vi "Teleop.vi"(10 "Match Info":T1={"Autonomous Elapsed Seconds"=0.0, "TeleOp Elapsed Seconds"=0.0, "Disabled Elapsed Seconds"=0.0, "Visited Autonomous"=FALSE, "Visited TeleOp"=FALSE, "Visited Disabled"=FALSE, "Autonomous Settings"={"Autonomous Style"=enum."Independent", "VI Refnum"=refnum}}, 11 "Call Context":T2) -> ()   [LabVIEW 2016]
doc: "This VI is called for each TeleOp packet received from the DS where the robot is not disabled. It is often used to read from the joysticks and update I/O or to update setpoints for timed control loops. It should complete and return within 20 milliseconds or it may miss DS packets."
uses:
  <vilib>/Rock Robotics/WPI/DriverStation/WPI_DriverStationDerivedRobotMode.ctl
  <vilib>/Rock Robotics/WPI/DriverStation/WPI_DriverStationMatch Info.ctl
  <vilib>/Rock Robotics/WPI/Solenoid/WPI_SolenoidValue.ctl
  <vilib>/Rock Robotics/WPI/ThirdParty/CanMotor/CTRLib-LV-TalonSRX/CTRE_CANTalonSRX_ControlMode.ctl
  <vilib>/Rock Robotics/WPI/Utilities/WPI_GetSetVariantRefNum.vi
  <vilib>/Rock Robotics/Network Tables/NT Write Boolean Array.vi
  <vilib>/Rock Robotics/Network Tables/NT Write Numeric Array.vi
  <vilib>/Rock Robotics/Network Tables/NT Read Boolean.vi
  <vilib>/Rock Robotics/Network Tables/NT Read Number.vi
  <vilib>/Rock Robotics/WPI/Solenoid/WPI_SolenoidSetEnum.vi
panel:
  out "Sample Slider 0":dbl(slide) scale=0.0..5.0
  out "Sample Boolean 1":bool
  out "Sample Boolean 0":bool
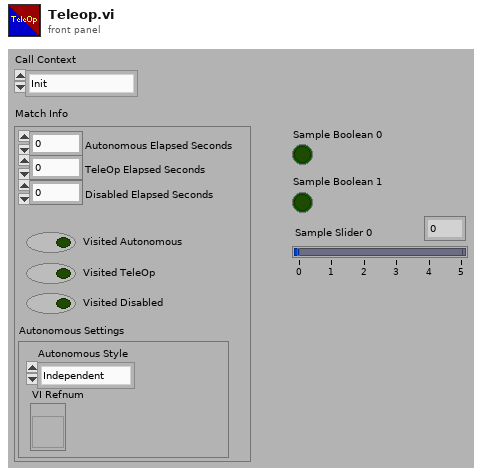
[diagram p1: front panel]
types:
  T1 = typedef "WPI_DriverStationMatch Info.ctl" = cluster{"Autonomous Elapsed Seconds":dbl, "TeleOp Elapsed Seconds":dbl, "Disabled Elapsed Seconds":dbl, "Visited Autonomous":bool, "Visited TeleOp":bool, "Visited Disabled":bool, "Autonomous Settings":cluster{"Autonomous Style":enum16{"Iterative", "Independent"}, "VI Refnum":refnum<vi>}}
  T2 = typedef "WPI_DriverStationDerivedRobotMode.ctl" = enum16{"Init", "Execute", "Stop"}
  T3 = typedef "CTRE_CANTalonSRX_ControlMode.ctl" = enum16{"Throttle (Duty-Cycle)", "Position Closed-Loop", "Velocity Closed-Loop", "Current Closed-Loop", "Voltage Compensation", "Slave Follower", "Motion Profile", "Motion Magic"}
  T4 = typedef "WPI_MotorControlDeviceRef.ctl" = cluster{"DeviceStatus":errorcluster, "Type":T5, "PWM":cluster{"PWM Channel":T6, "DeadBand":T7}, "CAN":cluster{"Device Number":u8, "SetOutput VI Ref":variant, "GetOutput VI Ref":variant, "Enable VI Ref":variant, "Disable VI Ref":variant, "Data":variant}, "Invert":bool}
  T5 = typedef "WPI_MotorControlType.ctl" = enum16{"PWM", "CAN"}
  T6 = typedef "FPGA_DIOPWMChannel.ctl" = enum8{"PWM 0", "PWM 1", "PWM 2", "PWM 3", "PWM 4", "PWM 5", "PWM 6", "PWM 7", "PWM 8", "PWM 9", "PWM MXP 0", "PWM MXP 1", "PWM MXP 2", "PWM MXP 3", "PWM MXP 4", "PWM MXP 5", "PWM MXP 6", "PWM MXP 7", "PWM MXP 8", "PWM MXP 9", "Invalid"}
  T7 = typedef "WPI_PWMDeadband.ctl" = cluster{"Name":string, "maxPositivePwm":i32, "minPositivePwm":i32, "centerPwm":i32, "maxNegativePwm":i32, "minNegativePwm":i32, "angularRange":u16}
  T8 = typedef "WPI_JoystickDevRef.ctl" = cluster{"Device":T9}
  T9 = typedef "WPI_JoystickDeviceEnum.ctl" = enum16{"USB 0", "USB 1", "USB 2", "USB 3", "USB 4", "USB 5"}
  T10 = cluster{"Axes[0]":dbl, "Axes[1]":dbl, "Axes[2]":dbl, "Axes[3]":dbl, "Axes[4]":dbl, "Axes[5]":dbl, "Axes[6]":dbl, "Axes[7]":dbl, "Axes[8]":dbl}
  T11 = cluster{"Buttons[0]":bool, "Buttons[1]":bool, "Buttons[2]":bool, "Buttons[3]":bool, "Buttons[4]":bool, "Buttons[5]":bool, "Buttons[6]":bool, "Buttons[7]":bool, "Buttons[8]":bool}
  T12 = cluster{"POVs[0]":i16, "POVs[1]":i16, "POVs[2]":i16, "POVs[3]":i16, "POVs[4]":i16, "POVs[5]":i16, "POVs[6]":i16, "POVs[7]":i16, "POVs[8]":i16}
  T13 = typedef "WPI_SolenoidDevRef.ctl" = cluster{"DevStatus":errorcluster, "Pneumatics Control Module":u8, "Forward Solenoid Channel":T14, "Reverse Solenoid Channel":T14}
  T14 = typedef "WPI_SolenoidChannel.ctl" = enum8{"Solenoid 0", "Solenoid 1", "Solenoid 2", "Solenoid 3", "Solenoid 4", "Solenoid 5", "Solenoid 6", "Solenoid 7", "Invalid"}
  T15 = typedef "WPI_SolenoidValue.ctl" = enum16{"Off", "On", "Forward", "Reverse"}
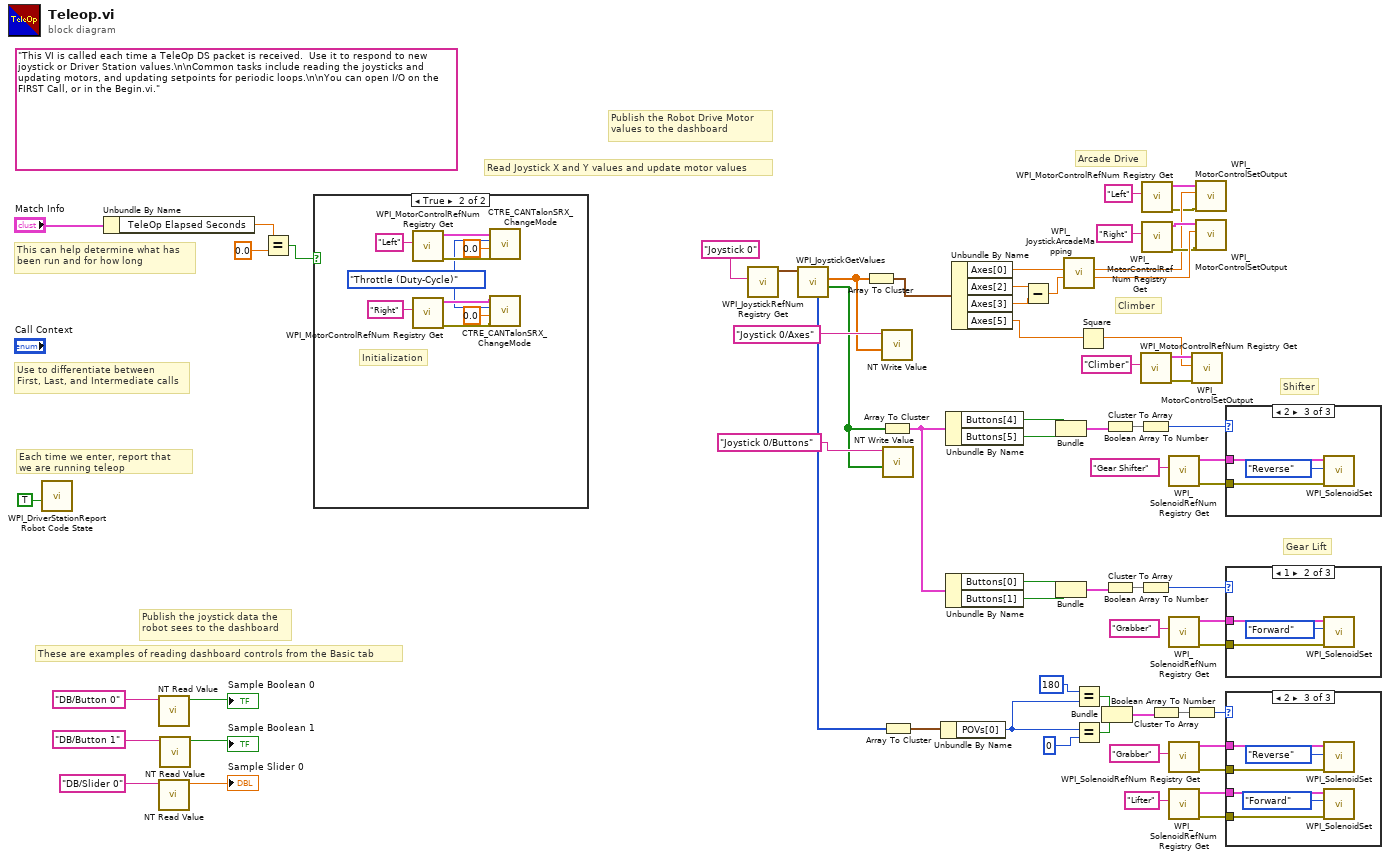
[diagram p0: block diagram]
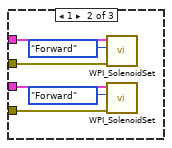
[diagram p3: hidden frame]
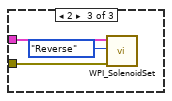
[diagram p5: hidden frame]
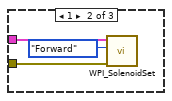
[diagram p7: hidden frame]
diagram:
  (unwired) "This VI is called each time a TeleOp DS packet is received.  Use it to respond to new joystick or Driver Station values.\n\nCommon tasks include reading the joysticks and updating motors, and updating setpoints for periodic loops.\n\nYou can open I/O on the FIRST Call, or in the Begin.vi."
  # "Gear Lift"
  # "Shifter"
  # "Climber"
  # "Arcade Drive"
  # "These are examples of reading dashboard controls from the Basic tab"
  # "Publish the Robot Drive Motor\nvalues to the dashboard"
  # "Publish the joystick data the\nrobot sees to the dashboard"
  # "Each time we enter, report that\nwe are running teleop"
  # "Use to differentiate between\nFirst, Last, and Intermediate calls"
  # "This can help determine what has\nbeen run and for how long"
  # "Read Joystick X and Y values and update motor values"
  n1 = call <vilib>:"WPI_DriverStationReport Robot Code State.vi"("TeleOp"=TRUE ("Autonomous")) -> ()  [unwired: 10 in, 1 out]
  n2 = Unbundle By Name("Match Info") -> ("TeleOp Elapsed Seconds"=w39:dbl)
  n3 = call-poly <vilib>:"NT Read Value.vi"("Name"="DB/Button 0" ("refnum name")) -> ("Boolean"=→"Sample Boolean 0":bool)  [unwired: 9 in, 1 out]
  n4 = call-poly <vilib>:"NT Read Value.vi"("Name"="DB/Slider 0" ("refnum name")) -> ("Numeric"=→"Sample Slider 0":dbl)  [unwired: 9 in, 1 out]
  n5 = call-poly <vilib>:"NT Read Value.vi"("Name"="DB/Button 1" ("refnum name")) -> ("Boolean"=→"Sample Boolean 1":bool)  [unwired: 9 in, 1 out]
  n6 = Equal?(x=w39, y=0.0) -> (x = y?=w38:bool)
  n7 = case shown="True" w38 {
    frame False {
    }
    frame True {
      w71 = CTRE_CANTalonSRX_ControlMode."Throttle (Duty-Cycle)" ("Talon SRX Control Mode")
      # "Initialization"
      n8 = call <vilib>:"WPI_MotorControlRefNum Registry Get.vi"("refnum name"="Left") -> ("error out"=w73:errorcluster, "MotorControlDevRef"=w74:T4)  [unwired: 9 in]
      n9 = call <vilib>:"WPI_MotorControlRefNum Registry Get.vi"("refnum name"="Right") -> ("error out"=w72:errorcluster, "MotorControlDevRef"=w75:T4)  [unwired: 9 in]
      n10 = call <vilib>:"CTRE_CANTalonSRX_ChangeMode.vi"("error in (no error)"=w73, "Output"=0.0, "Talon SRX Control Mode"=w71, "CAN Talon SRX Ref"=w74) -> ()  [unwired: 6 in, 2 out]
      n11 = call <vilib>:"CTRE_CANTalonSRX_ChangeMode.vi"("error in (no error)"=w72, "Output"=0.0, "Talon SRX Control Mode"=w71, "CAN Talon SRX Ref"=w75) -> ()  [unwired: 6 in, 2 out]
    }
  }
  n12 = call <vilib>:"WPI_JoystickRefNum Registry Get.vi"("refnum name"="Joystick 0") -> ("JoystickDevRef"=w66:T8)  [unwired: 1 in, 9 out]
  n13 = call <vilib>:"WPI_JoystickGetValues.vi"("JoystickDevRef"=w66) -> ("Buttons"=w56:bool[], "Axes"=w54:dbl[], "POVs"=w55:i16[])  [unwired: 6 in, 2 out]
  n14 = Array To Cluster(array=w54) -> (cluster=w53:T10)
  n15 = call-poly <vilib>:"NT Write Value.vi"("Numeric Array"=w54, "Name"="Joystick 0/Axes") -> ()  [unwired: 9 in, 1 out]
  n16 = Array To Cluster(array=w56) -> (cluster=w20:T11)
  n17 = call-poly <vilib>:"NT Write Value.vi"("Boolean Array"=w56, "Name"="Joystick 0/Buttons") -> ()  [unwired: 9 in, 1 out]
  n18 = Array To Cluster(array=w55) -> (cluster=w52:T12)
  n19 = Unbundle By Name(w52) -> ("POVs[0]"=w23:i16)
  n20 = Unbundle By Name(w20) -> ("Buttons[4]"=w31:bool, "Buttons[5]"=w30:bool)
  n21 = Unbundle By Name(w20) -> ("Buttons[0]"=w13:bool, "Buttons[1]"=w12:bool)
  n22 = Unbundle By Name(w53) -> ("Axes[0]"=w37:dbl, "Axes[2]"=w49:dbl, "Axes[3]"=w48:dbl, "Axes[5]"=w33:dbl)
  n23 = Subtract(x=w49, y=w48) -> (x-y=w47:dbl)
  n24 = Bundle("Buttons[4]"=w31, "Buttons[5]"=w30) -> (w29:cluster{"Buttons[4]":bool, "Buttons[5]":bool})  [unwired: 1 in]
  n25 = Bundle("Buttons[0]"=w13, "Buttons[1]"=w12) -> (w19:cluster{"Buttons[0]":bool, "Buttons[1]":bool})  [unwired: 1 in]
  n26 = call <vilib>:"WPI_JoystickArcadeMapping.vi"("Y axis value"=w47, "X axis value"=w37) -> ("Right Motor Value"=w46:dbl, "Left Motor Value"=w43:dbl)  [unwired: 8 in]
  n27 = Equal?(x=i16 180, y=w23) -> (x = y?=w5:bool)
  n28 = Equal?(x=w23, y=i16 0) -> (x = y?=w4:bool)
  n29 = Square(x=w33) -> (x^2=w32:dbl)
  n30 = Bundle(w5, w4) -> (w11:cluster{bool, bool})  [unwired: 1 in]
  n31 = Cluster To Array(cluster=w29) -> (array=w28:bool[])
  n32 = Cluster To Array(cluster=w19) -> (array=w18:bool[])
  n33 = call <vilib>:"WPI_MotorControlRefNum Registry Get.vi"("refnum name"="Climber") -> ("error out"=w34:errorcluster, "MotorControlDevRef"=w35:T4)  [unwired: 9 in]
  n34 = Boolean Array To Number(Boolean array=w28) -> (number=w27:u32)
  n35 = Boolean Array To Number(Boolean array=w18) -> (number=w17:u32)
  n36 = call <vilib>:"WPI_MotorControlRefNum Registry Get.vi"("refnum name"="Left") -> ("error out"=w41:errorcluster, "MotorControlDevRef"=w42:T4)  [unwired: 9 in]
  n37 = call <vilib>:"WPI_MotorControlRefNum Registry Get.vi"("refnum name"="Right") -> ("error out"=w44:errorcluster, "MotorControlDevRef"=w45:T4)  [unwired: 9 in]
  n38 = Cluster To Array(cluster=w11) -> (array=w10:bool[])
  n39 = call <vilib>:"WPI_SolenoidRefNum Registry Get.vi"("refnum name"="Gear Shifter") -> ("error out"=w25:errorcluster, "SolenoidDevRef"=w26:T13)  [unwired: 9 in]
  n40 = call <vilib>:"WPI_SolenoidRefNum Registry Get.vi"("refnum name"="Grabber") -> ("error out"=w15:errorcluster, "SolenoidDevRef"=w16:T13)  [unwired: 9 in]
  n41 = call <vilib>:"WPI_SolenoidRefNum Registry Get.vi"("refnum name"="Grabber") -> ("error out"=w7:errorcluster, "SolenoidDevRef"=w8:T13)  [unwired: 9 in]
  n42 = call <vilib>:"WPI_SolenoidRefNum Registry Get.vi"("refnum name"="Lifter") -> ("error out"=w2:errorcluster, "SolenoidDevRef"=w1:T13)  [unwired: 9 in]
  n43 = Boolean Array To Number(Boolean array=w10) -> (number=w9:u32)
  n44 = call <vilib>:"WPI_MotorControlSetOutput.vi"("error in (no error)"=w34, "Output"=w32, "MotorControlDevRef"=w35) -> ()  [unwired: 6 in, 3 out]
  n45 = call <vilib>:"WPI_MotorControlSetOutput.vi"("error in (no error)"=w41, "Output"=w43, "MotorControlDevRef"=w42) -> ()  [unwired: 6 in, 3 out]
  n46 = call <vilib>:"WPI_MotorControlSetOutput.vi"("error in (no error)"=w44, "Output"=w46, "MotorControlDevRef"=w45) -> ()  [unwired: 6 in, 3 out]
  n47 = case shown="2" w27 {
    tunnel: w26 -> [_ w79 w82]
    tunnel: w25 -> [_ w78 w81]
    frame 0, Default {
    }
    frame 1 {
      n48 = call-poly <vilib>:"WPI_SolenoidSet.vi"("error in (no error)"=w78, "Value"=WPI_SolenoidValue."Forward", "SolenoidDevRef"=w79) -> ()  [unwired: 7 in, 2 out]
    }
    frame 2 {
      n49 = call-poly <vilib>:"WPI_SolenoidSet.vi"("error in (no error)"=w81, "Value"=WPI_SolenoidValue."Reverse", "SolenoidDevRef"=w82) -> ()  [unwired: 7 in, 2 out]
    }
  }
  n50 = case shown="1" w17 {
    tunnel: w16 -> [_ w85 w88]
    tunnel: w15 -> [_ w84 w87]
    frame 0, Default {
    }
    frame 1 {
      n51 = call-poly <vilib>:"WPI_SolenoidSet.vi"("error in (no error)"=w84, "Value"=WPI_SolenoidValue."Forward", "SolenoidDevRef"=w85) -> ()  [unwired: 7 in, 2 out]
    }
    frame 2 {
      n52 = call-poly <vilib>:"WPI_SolenoidSet.vi"("error in (no error)"=w87, "Value"=WPI_SolenoidValue."Reverse", "SolenoidDevRef"=w88) -> ()  [unwired: 7 in, 2 out]
    }
  }
  n53 = case shown="2" w9 {
    tunnel: w8 -> [_ w94 w100]
    tunnel: w7 -> [_ w93 w99]
    tunnel: w1 -> [_ w91 w97]
    tunnel: w2 -> [_ w92 w96]
    frame 0, Default {
    }
    frame 1 {
      n54 = call-poly <vilib>:"WPI_SolenoidSet.vi"("error in (no error)"=w93, "Value"=WPI_SolenoidValue."Forward", "SolenoidDevRef"=w94) -> ()  [unwired: 7 in, 2 out]
      n55 = call-poly <vilib>:"WPI_SolenoidSet.vi"("error in (no error)"=w92, "Value"=WPI_SolenoidValue."Forward", "SolenoidDevRef"=w91) -> ()  [unwired: 7 in, 2 out]
    }
    frame 2 {
      n56 = call-poly <vilib>:"WPI_SolenoidSet.vi"("error in (no error)"=w99, "Value"=WPI_SolenoidValue."Reverse", "SolenoidDevRef"=w100) -> ()  [unwired: 7 in, 2 out]
      n57 = call-poly <vilib>:"WPI_SolenoidSet.vi"("error in (no error)"=w96, "Value"=WPI_SolenoidValue."Forward", "SolenoidDevRef"=w97) -> ()  [unwired: 7 in, 2 out]
    }
  }
